vi "exec.vi"(8 "error in (no error)":errorcluster, 10 "context":refnum<class "IContextThisComponent.lvclass">, 11 "GoToStandby in":refnum<class "standby.lvclass">) -> (0 "error out":errorcluster, 2 "context 2":refnum<class "IContextThisComponent.lvclass">, 3 "GoToStandby out":refnum<class "standby.lvclass">)   [LabVIEW 2016, in "Commands.lvlib" / "standby.lvclass"]
uses:
  standby.lvclass
  IContextThisComponent/IContextThisComponent.lvclass
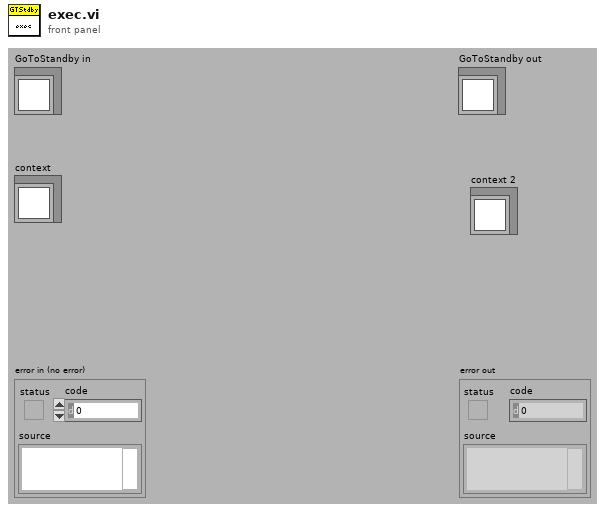
[diagram p1: front panel]
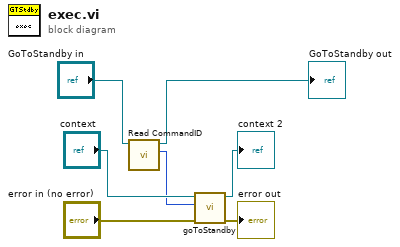
[diagram p0: block diagram]
diagram:
  n1 = call-dynamic "Read CommandID.vi"("Command in"="GoToStandby in") -> ("CommandID"=w1:i32, "Command out"=→"GoToStandby out":refnum<class "standby.lvclass">)  [unwired: 8 in, 1 out]
  n2 = call-dynamic "goToStandby.vi"("error in (no error)"="error in (no error)", "CommandID"=w1, "IContextThisComponent in"="context") -> ("error out"=→"error out":errorcluster, "IContextThisComponent out"=→"context 2":refnum<class "IContextThisComponent.lvclass">)  [unwired: 7 in]
